vi "Valid_Path.vi"(1 "Filename":path) -> (0 "Valid Path?":bool)   [LabVIEW 2018]
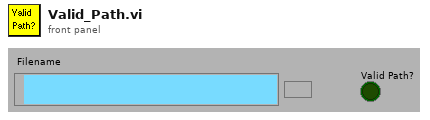
[diagram p1: front panel]
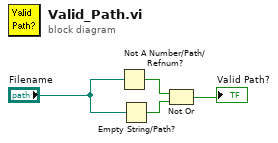
[diagram p0: block diagram]
diagram:
  n1 = Not A Number/Path/Refnum?(number/path/refnum="Filename") -> (NaN/Path/Refnum?=w2:bool)
  n2 = Empty String/Path?(string/path="Filename") -> (empty?=w3:bool)
  n3 = Not Or(1:w3, 2:w2) -> (0:→"Valid Path?":bool)
